vi "SD Read Rarely.vi"   [LabVIEW 2013]
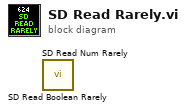
[diagram p0: block diagram]
diagram:
  n1 = call "SD Read Boolean Rarely.vi"() -> ()  [unwired: 11 in, 1 out]
  n2 = call "SD Read Num Rarely.vi"() -> ()  [unwired: 11 in, 1 out]
